vi "Update_2layer_Wx_FPGA.vi"(0 "Target_OutX":fxp<+/-,32,8>, 1 "2layer_OutX":fxp<+/-,32,8>, 2 "Learning rate":fxp<+/-,32,8>, 3 "Array_Out_hx":fxp<+/-,32,8>[](array[numeric])=[0.0, 0.0, 0.0, 0.0], 4 "Weights_2layer":fxp<+/-,32,8>[](array[numeric])=[0.0, 0.0, 0.0, 0.0]) -> (5 "Weights_2layer_updated":fxp<+/-,32,8>[](array[numeric]))   [LabVIEW 2016]
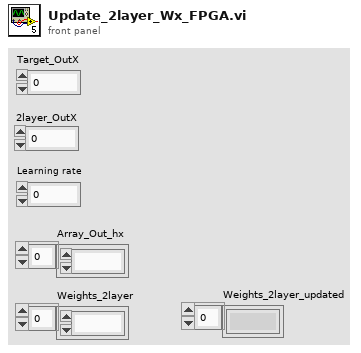
[diagram p1: front panel]
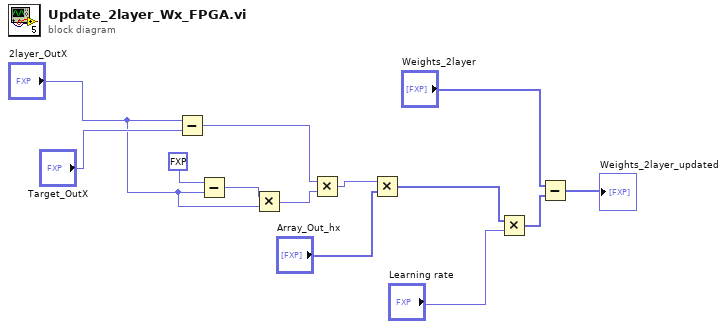
[diagram p0: block diagram]
diagram:
  n1 = Subtract(x="2layer_OutX", y="Target_OutX") -> (x-y=w10:fxp<+/-,32,8>)
  n2 = Subtract(x=fxp<+,32,8> 1.0, y="2layer_OutX") -> (x-y=w12:fxp<+/-,32,8>)
  n3 = Multiply(x=w12, y="2layer_OutX") -> (x*y=w9:fxp<+/-,32,8>)
  n4 = Multiply(x=w10, y=w9) -> (x*y=w5:fxp<+/-,32,8>)
  n5 = Multiply(x=w5, y="Array_Out_hx") -> (x*y=w3:fxp<+/-,64,16>[])
  n6 = Multiply(x=w3, y="Learning rate") -> (x*y=w8:fxp<+/-,32,8>[])
  n7 = Subtract(x="Weights_2layer", y=w8) -> (x-y=→"Weights_2layer_updated":fxp<+/-,32,8>[])
